vi "Pot Data.vi"(7 "Read//Write":T1, 11 "Voltage In":dbl) -> (3 "Voltage Out":dbl)   [LabVIEW 2018]
uses:
  Type Defs/Read Write.ctl
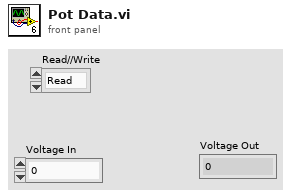
[diagram p1: front panel]
types:
  T1 = typedef "Read Write.ctl" = enum16{"Read", "Write"}
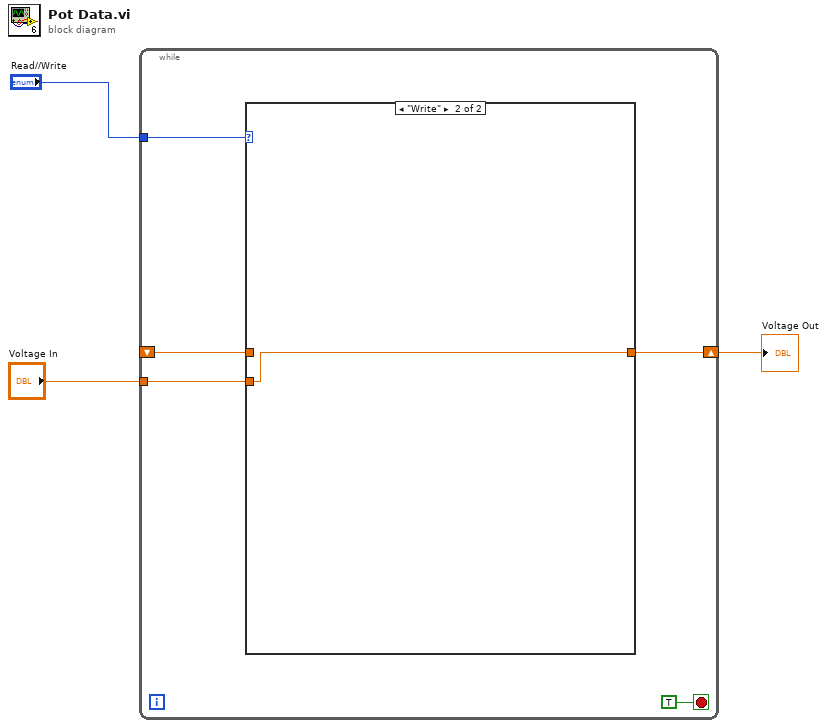
[diagram p0: block diagram]
diagram:
  n1 = while {
    tunnel: "Read//Write" -> [w7]
    shift-right: [w5] -> w2
    shift-left: _ -> [w4]
    tunnel: "Voltage In" -> [w6]
    stop <- TRUE stop-if-true
    n2 = case shown="\"Write\"" w7 {
      tunnel: w6 -> [_ w10]
      tunnel: [w9 w10] -> w5
      tunnel: w4 -> [w9 _]
      frame "Read", Default {
      }
      frame "Write" {
      }
    }
  }
  "Voltage Out" <- w2
